vi "Call Import With Path.vi"(8 "error in (no error)":errorcluster, 10 "Path":path, 11 "Node Ptr":u64) -> (0 "error out":errorcluster, 3 "Node Ptr out":u64)   [LabVIEW 2017, in "SLSC Switch Import Export Unit Tests.lvclass"]
uses:
  SLSC Switch Import Export Unit Tests.lvclass
  System Explorer/Import Configuration RTM.vi
  System Explorer/SLSC Switch System Explorer.lvlib
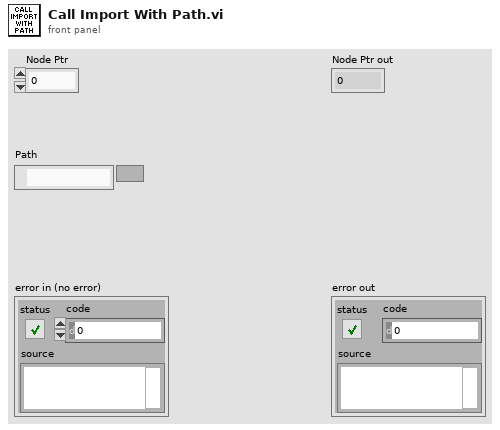
[diagram p1: front panel]
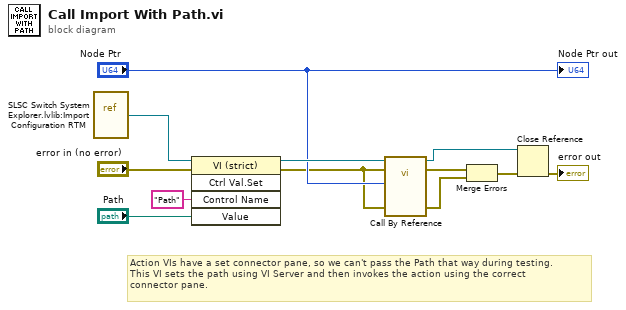
[diagram p0: block diagram]
diagram:
  # "Action VIs have a set connector pane, so we can't pass the Path that way during testing.\nThis VI sets the path using VI Server and then invokes the action using the correct\nconnector pane."
  n1 = vi-ref "SLSC Switch System Explorer.lvlib:Import Configuration RTM.vi"() -> (w12:refnum<vi>)
  n2 = invoke class="VI (strict)" method="Ctrl Val.Set"(reference=w12, error in="error in (no error)", "Control Name"="Path", "Value"="Path") -> (reference out=w10:refnum<vi>, error out=w6:errorcluster)  [unwired: 1 in, 3 out]
  n3 = call-by-ref "?"(reference=w10, error in=w6, 8:"error in (no error)"=w6, "Node Ptr"="Node Ptr") -> (reference out=w2:refnum<vi>, error out=w5:errorcluster, 0:"error out"=w4:errorcluster)  [unwired: 9 in]
  n4 = Merge Errors(w5, w4) -> (w3:errorcluster)
  n5 = Close Reference(reference=w2, error in (no error)=w3) -> (error out=→"error out":errorcluster)
  "Node Ptr out" <- "Node Ptr"
